vi "内置参数设置.vi"() -> ()   [LabVIEW 2016, in "斯坦道CODMn新电路板.lvlib"]
uses:
  <vilib>/Utility/miscctls.llb/LVPointTypeDef.ctl
panel:
  in  "滴定延时时间:\n(单位:毫秒)":u16
  in  "斜率阈值:":dbl
  in  "阀配置:":u8(ring) items=["三通阀", "排阀"]
  in  "AB跨度告警值:":u16
  in  "B值告警上限值:":u16
  in  "B值范围:":u16
  in  "A值告警上限值:":u16
  in  "A值范围:":u16
  in  "是否存在液位检测板:":u16(ring) items=["否", "是"]
  in  "检出限(mg/L):":dbl
  in  "测量精度(mg/L):":dbl
  in  "ILimitDown":dbl
  in  "ILimitUp:":dbl
  in  "K d:":dbl
  in  "K i:":dbl
  in  "K p:":dbl
  in  "加热超时时间:(单位:秒)":dbl
  in  "告警温度:":dbl
  in  "加热温度:  校准参数":dbl
  in  "运行速度:  (修改需要重启)":u16
  in  "偏心轮: 校准参数":dbl
  in  "注射泵加热超时时间(s):":u16
  in  "注射泵保温温度H:":u8
  in  "注射泵\n保温温度L:":u8
  in  "传感器阈值:":u16
  in  "纯水通道:":u16
  in  "滴定速度:":u16
  in  "出样速度:":u16
  in  "进样速度:":u16
  in  "阀数量:":u8(ring) items=["9通"=9, "12通"=12]
  in  "注射泵型号":u8(ring) items=["TECAN", "润泽", "旋转阀"]
  in  "阈值(高→低)(mg/L):":dbl
  in  "阈值(低→高)(mg/L):":dbl
  in  "检测下限(mg/L):":dbl
  in  "检测上限(mg/L):":dbl
  in  "关闭":bool
  in  "保存":bool
  in  "读取":bool
  # "仪器内部参数设置"
  # "~"
  # "~"
  # "~"
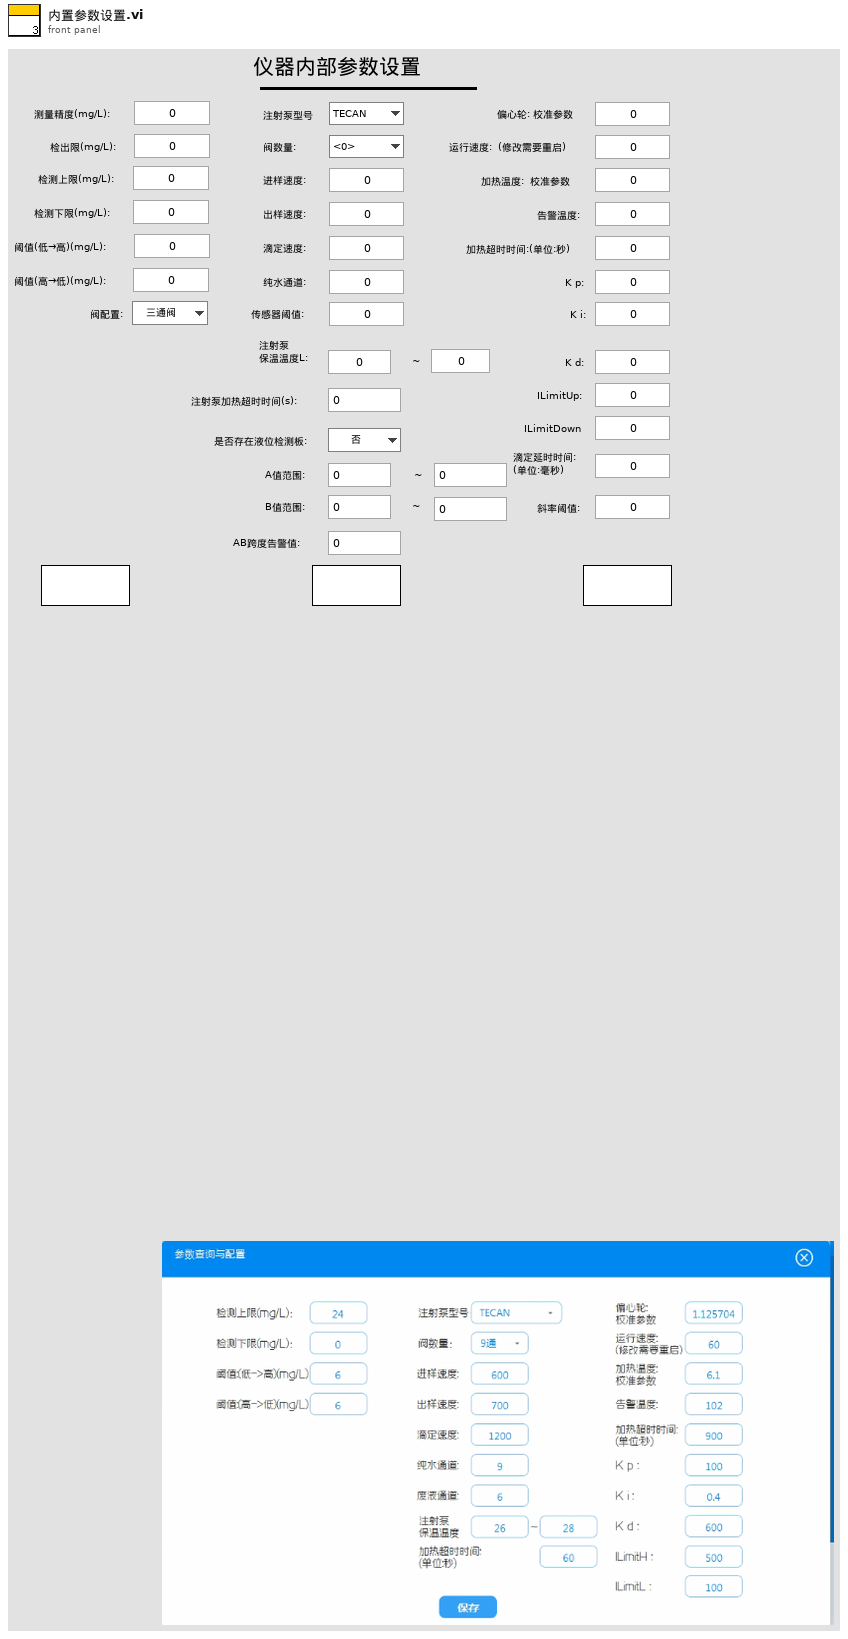
[diagram p1: front panel]
types:
  T1 = typedef "LVPointTypeDef.ctl" = cluster{"Horizontal":i16, "Vertical":i16}
  T2 = cluster{"偏心轮校准参数":dbl, "运行速度(修改需要重启)":u16, "加热温度(校准参数) ":dbl, "告警温度":dbl, "加热超时时间:(单位/秒)":dbl, "K p":dbl, "K i":dbl, "K d":dbl, "ILimitUp":dbl, "ILimitDown":dbl}
  T3 = cluster{"泵类型":u8, "阀数量":u8, "纯水通道":u16, "废液通道":u8, "进样速度":u16, "出样速度":u16, "滴定速度":u16, "注射泵保温温度L":u8, "注射泵保温温度H":u8, "注射泵加热超时时间":u16, "是否存在液位检测板":u16, "A值告警下限值":u16, "A值告警上限值":u16, "B值告警下限值":u16, "B值告警上限值":u16, "AB跨度告警值":u16, "阀配置:":u8, "滴定等待时间":u16, "滴定吸光度斜率":dbl, "传感器阈值":u16}
  T4 = cluster{"检出限":dbl, "测量精度":dbl, "上限":dbl, "下限":dbl, "阈值（低->高）":dbl, "阈值（高->低）":dbl}
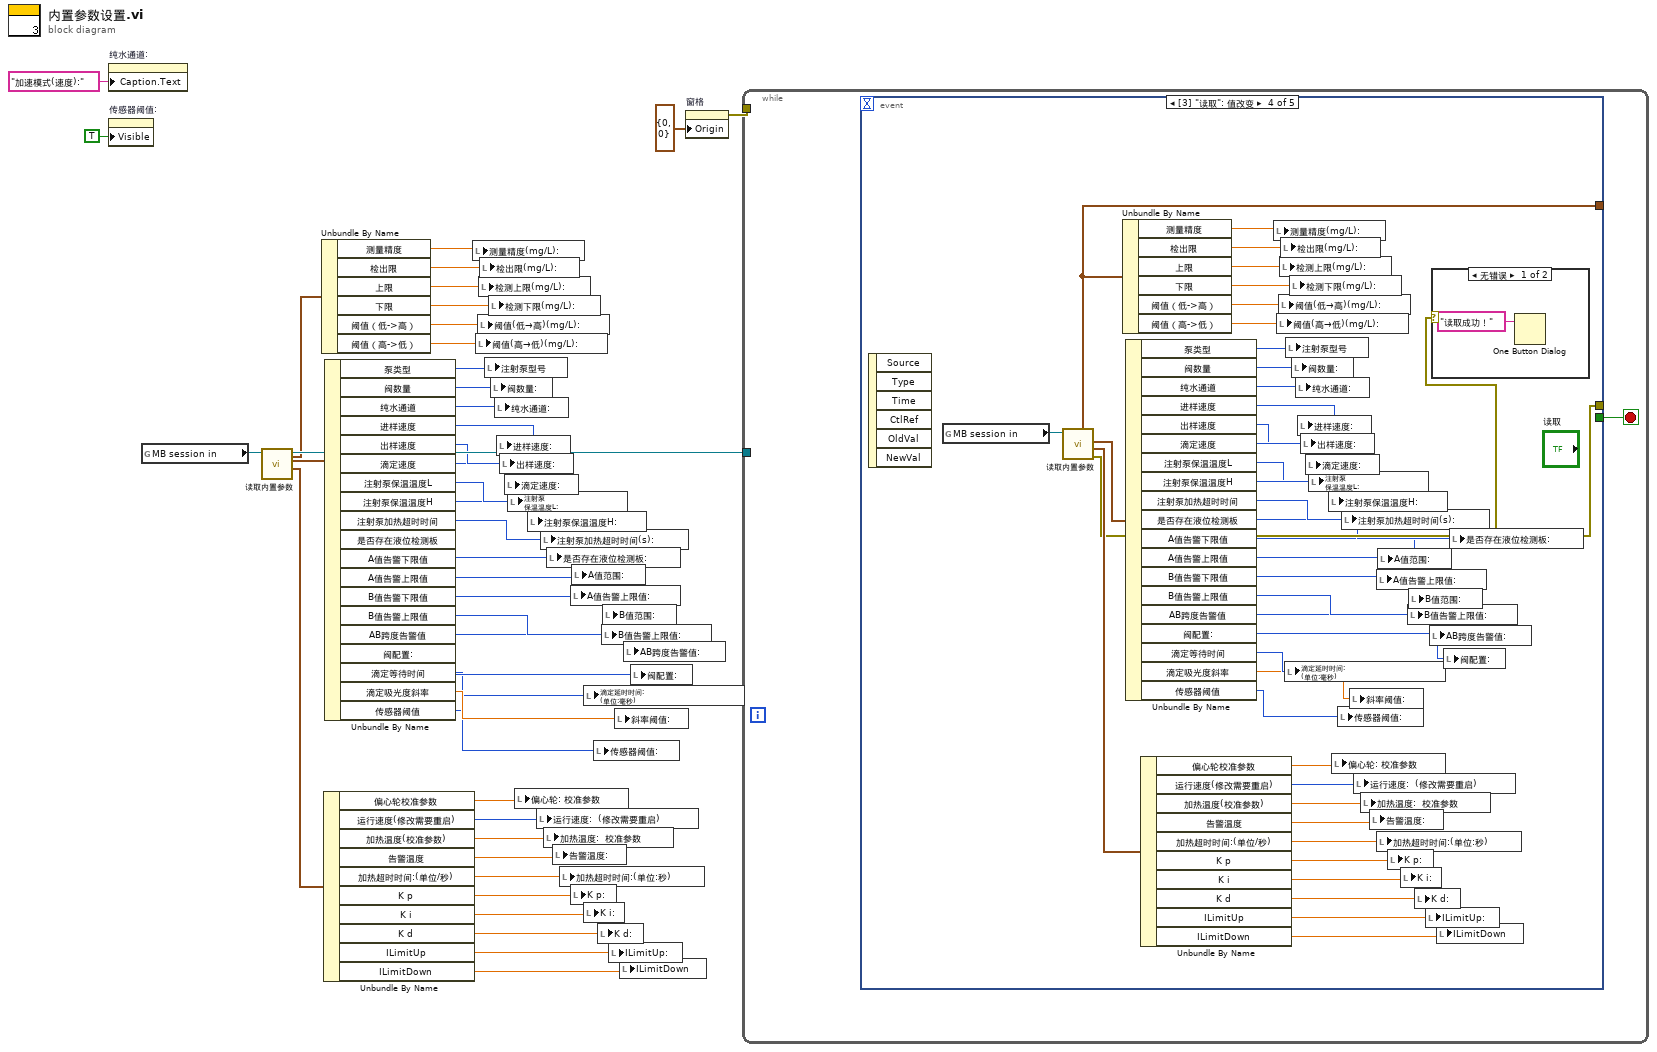
[diagram p0: block diagram]
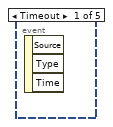
[diagram p2: hidden frame]
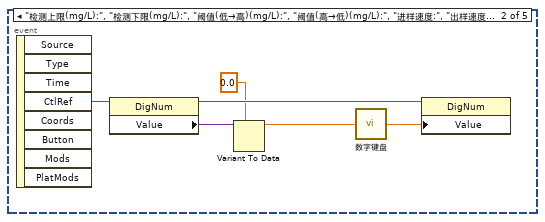
[diagram p3: hidden frame]
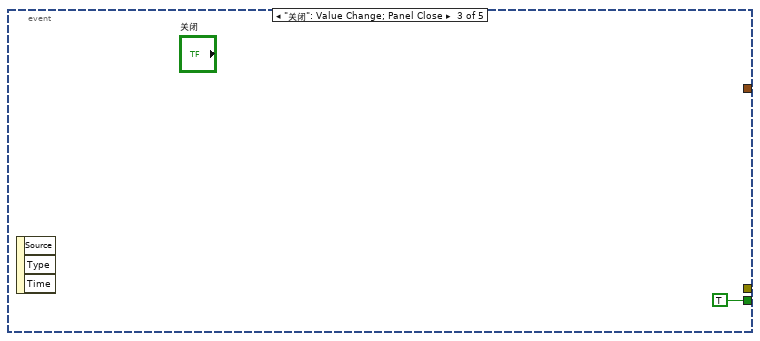
[diagram p4: hidden frame]
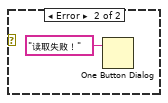
[diagram p5: hidden frame]
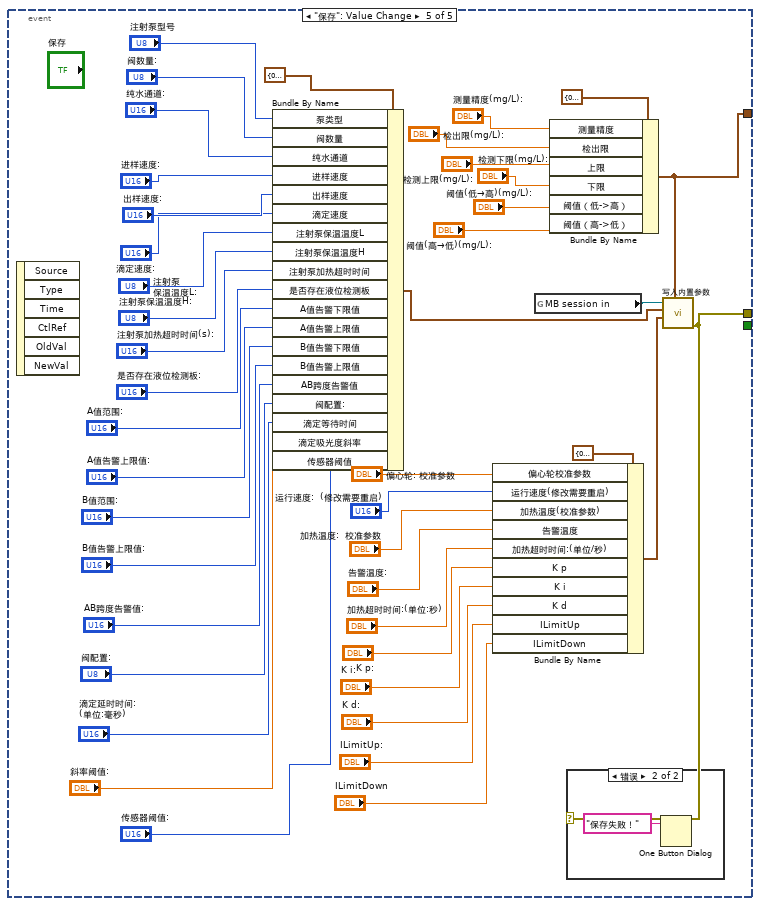
[diagram p6: hidden frame]
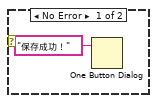
[diagram p7: hidden frame]
diagram:
  n1 = property on="纯水通道:" class="DigNum (严格)"("Caption.Text"="加速模式(速度):" ("标题.文本")) -> ()  [unwired: 2 in, 2 out]
  n2 = property on="传感器阈值:" class="DigNum (严格)"("Visible"=TRUE ("可见")) -> ()  [unwired: 2 in, 2 out]
  n3 = global read "VARCODMn全局变量.vi" "MB session in"() -> (w42:refnum<class "MB_Master.lvclass">)
  n4 = call "读取内置参数.vi"("MB session in"=w42) -> ("float"=w39:T2, "外设配置"=w40:T3, "MB session out"=w41:refnum<class "MB_Master.lvclass">, "量程参数读取"=w6:T4)  [unwired: 6 in, 1 out]
  n5 = Unbundle By Name(w6) -> ("测量精度"=w38:dbl, "检出限"=w37:dbl, "上限"=w36:dbl, "下限"=w35:dbl, "阈值（低->高）"=w34:dbl, "阈值（高->低）"=w33:dbl)
  n6 = Unbundle By Name(w39) -> ("偏心轮校准参数"=w23:dbl, "运行速度(修改需要重启)"=w22:u16, "加热温度(校准参数)"=w21:dbl, "告警温度"=w20:dbl, "加热超时时间:(单位/秒)"=w19:dbl, "K p"=w18:dbl, "K i"=w17:dbl, "K d"=w16:dbl, "ILimitUp"=w15:dbl, "ILimitDown"=w14:dbl)
  n7 = Unbundle By Name(w40) -> ("泵类型"=w32:u8, "阀数量"=w31:u8, "纯水通道"=w30:u16, "进样速度"=w29:u16, "出样速度"=w28:u16, "滴定速度"=w27:u16, "注射泵保温温度L"=w26:u8, "注射泵保温温度H"=w25:u8, "注射泵加热超时时间"=w24:u16, "是否存在液位检测板"=w13:u16, "A值告警下限值"=w12:u16, "A值告警上限值"=w11:u16, "B值告警下限值"=w10:u16, "B值告警上限值"=w9:u16, "AB跨度告警值"=w8:u16, "阀配置:"=w7:u8, "滴定等待时间"=w4:u16, "滴定吸光度斜率"=w5:dbl, "传感器阈值"=w1:u16)
  n8 = local write "测量精度(mg/L):"(w38) -> ()
  n9 = local write "阈值(高→低)(mg/L):"(w33) -> ()
  n10 = local write "阈值(低→高)(mg/L):"(w34) -> ()
  n11 = local write "检测上限(mg/L):"(w36) -> ()
  n12 = local write "检出限(mg/L):"(w37) -> ()
  n13 = local write "注射泵型号"(w32) -> ()
  n14 = local write "检测下限(mg/L):"(w35) -> ()
  n15 = local write "阀数量:"(w31) -> ()
  n16 = local write "纯水通道:"(w30) -> ()
  n17 = local write "进样速度:"(w29) -> ()
  n18 = local write "出样速度:"(w28) -> ()
  n19 = local write "滴定速度:"(w27) -> ()
  n20 = local write "注射泵\n保温温度L:"(w26) -> ()
  n21 = local write "偏心轮: 校准参数"(w23) -> ()
  n22 = local write "注射泵保温温度H:"(w25) -> ()
  n23 = local write "运行速度:  (修改需要重启)"(w22) -> ()
  n24 = local write "注射泵加热超时时间(s):"(w24) -> ()
  n25 = local write "加热温度:  校准参数"(w21) -> ()
  n26 = local write "是否存在液位检测板:"(w13) -> ()
  n27 = local write "告警温度:"(w20) -> ()
  n28 = local write "加热超时时间:(单位:秒)"(w19) -> ()
  n29 = local write "A值告警上限值:"(w11) -> ()
  n30 = local write "K p:"(w18) -> ()
  n31 = local write "A值范围:"(w12) -> ()
  n32 = local write "滴定延时时间:\n(单位:毫秒)"(w4) -> ()
  n33 = local write "K i:"(w17) -> ()
  n34 = local write "传感器阈值:"(w1) -> ()
  n35 = local write "K d:"(w16) -> ()
  n36 = local write "B值告警上限值:"(w9) -> ()
  n37 = local write "B值范围:"(w10) -> ()
  n38 = local write "ILimitUp:"(w15) -> ()
  n39 = local write "斜率阈值:"(w5) -> ()
  n40 = local write "ILimitDown"(w14) -> ()
  n41 = local write "AB跨度告警值:"(w8) -> ()
  n42 = local write "阀配置:"(w7) -> ()
  n43 = property on="窗格" class="Pane"("Origin"=T1 {"Horizontal"=0, "Vertical"=0} ("原点")) -> (error out=w43:errorcluster)  [unwired: 2 in, 1 out]
  n44 = while {
    tunnel: w43 -> [_]
    tunnel: w41 -> [_]
    stop <- w45 stop-if-true
    n45 = event shown="[3] \"读取\": 值改变" {
      selector: _ -> [_ _ _ _ _]
      dyn-events: _ -> [_ _ _ _ _]
      timeout: _ -> [_ _ _ _ _]
      tunnel: [_ _ TRUE _ _] -> w45
      tunnel: [_ _ _ w64 w109] -> _
      tunnel: [_ _ _ w56 w100] -> _
      event Timeout {
        n46 = event-data() -> ()  [unwired: 1 in, 3 out]
      }
      event "检测上限(mg/L):", "检测下限(mg/L):", "阈值(低→高)(mg/L):", "阈值(高→低)(mg/L):", "进样速度:", "出样速度:", "滴定速度:", "纯水通道:", "传感器阈值:", "注射泵\n保温温度L:", "注射泵保温温度H:", "注射泵加热超时时间(s):", "偏心轮: 校准参数", "运行速度:  (修改需要重启)", "告警温度:", "加热温度:  校准参数", "K p:", "K i:", "K d:", "ILimitUp:", "ILimitDown", "测量精度(mg/L):", "检出限(mg/L):", "A值范围:", "A值告警上限值:", "B值范围:", "B值告警上限值:", "AB跨度告警值:", "斜率阈值:", "滴定延时时间:\n(单位:毫秒)": Mouse Down {
        n47 = event-data() -> ("CtlRef"=w51:refnum<vi>)  [unwired: 1 in, 7 out]
        n48 = property class="DigNum"(reference=w51) -> (reference out=w50:refnum<vi>, "Value"=w48:variant)  [unwired: 1 in, 1 out]
        n49 = Variant To Data(type=0.0 ("OldNumber"), Variant=w48) -> (data=w46:dbl)  [unwired: 1 in, 1 out]
        n50 = call "数字键盘.vi"("OldNumber"=w46) -> ("NewNumber"=w49:dbl)
        n51 = property class="DigNum"(reference=w50, "Value"=w49) -> ()  [unwired: 1 in, 2 out]
      }
      event "关闭": Value Change; Panel Close {
        n52 = event-data() -> ()  [unwired: 1 in, 3 out]
      }
      event "读取": Value Change {
        n53 = event-data() -> ()  [unwired: 1 in, 6 out]
        n54 = global read "VARCODMn全局变量.vi" "MB session in"() -> (w65:refnum<class "MB_Master.lvclass">)
        n55 = call "读取内置参数.vi"("MB session in"=w65) -> ("error out"=w64:errorcluster, "float"=w67:T2, "外设配置"=w66:T3, "量程参数读取"=w56:T4)  [unwired: 6 in, 1 out]
        n56 = Unbundle By Name(w56) -> ("测量精度"=w68:dbl, "检出限"=w69:dbl, "上限"=w70:dbl, "下限"=w71:dbl, "阈值（低->高）"=w72:dbl, "阈值（高->低）"=w73:dbl)
        n57 = Unbundle By Name(w66) -> ("泵类型"=w74:u8, "阀数量"=w75:u8, "纯水通道"=w76:u16, "进样速度"=w77:u16, "出样速度"=w78:u16, "滴定速度"=w79:u16, "注射泵保温温度L"=w80:u8, "注射泵保温温度H"=w81:u8, "注射泵加热超时时间"=w82:u16, "是否存在液位检测板"=w63:u16, "A值告警下限值"=w62:u16, "A值告警上限值"=w61:u16, "B值告警下限值"=w60:u16, "B值告警上限值"=w59:u16, "AB跨度告警值"=w58:u16, "阀配置:"=w57:u8, "滴定等待时间"=w55:u16, "滴定吸光度斜率"=w54:dbl, "传感器阈值"=w53:u16)
        n58 = Unbundle By Name(w67) -> ("偏心轮校准参数"=w83:dbl, "运行速度(修改需要重启)"=w84:u16, "加热温度(校准参数)"=w85:dbl, "告警温度"=w86:dbl, "加热超时时间:(单位/秒)"=w87:dbl, "K p"=w88:dbl, "K i"=w89:dbl, "K d"=w90:dbl, "ILimitUp"=w91:dbl, "ILimitDown"=w92:dbl)
        n59 = local write "测量精度(mg/L):"(w68) -> ()
        n60 = local write "阈值(高→低)(mg/L):"(w73) -> ()
        n61 = local write "阈值(低→高)(mg/L):"(w72) -> ()
        n62 = local write "检测上限(mg/L):"(w70) -> ()
        n63 = local write "检出限(mg/L):"(w69) -> ()
        n64 = local write "滴定延时时间:\n(单位:毫秒)"(w55) -> ()
        n65 = local write "注射泵型号"(w74) -> ()
        n66 = local write "检测下限(mg/L):"(w71) -> ()
        n67 = local write "阀数量:"(w75) -> ()
        n68 = local write "纯水通道:"(w76) -> ()
        n69 = local write "进样速度:"(w77) -> ()
        n70 = local write "出样速度:"(w78) -> ()
        n71 = local write "滴定速度:"(w79) -> ()
        n72 = local write "注射泵\n保温温度L:"(w80) -> ()
        n73 = local write "注射泵保温温度H:"(w81) -> ()
        n74 = local write "偏心轮: 校准参数"(w83) -> ()
        n75 = local write "传感器阈值:"(w53) -> ()
        n76 = local write "注射泵加热超时时间(s):"(w82) -> ()
        n77 = local write "斜率阈值:"(w54) -> ()
        n78 = local write "运行速度:  (修改需要重启)"(w84) -> ()
        n79 = local write "加热温度:  校准参数"(w85) -> ()
        n80 = local write "告警温度:"(w86) -> ()
        n81 = local write "A值告警上限值:"(w61) -> ()
        n82 = local write "加热超时时间:(单位:秒)"(w87) -> ()
        n83 = local write "A值范围:"(w62) -> ()
        n84 = local write "K p:"(w88) -> ()
        n85 = local write "K i:"(w89) -> ()
        n86 = local write "B值告警上限值:"(w59) -> ()
        n87 = local write "B值范围:"(w60) -> ()
        n88 = local write "K d:"(w90) -> ()
        n89 = local write "ILimitUp:"(w91) -> ()
        n90 = local write "AB跨度告警值:"(w58) -> ()
        n91 = case shown="无错误" w64 {
          frame No Error {
            n92 = One Button Dialog(message="读取成功！" ("消息")) -> ()  [unwired: 1 in, 1 out]
          }
          frame Error {
            n93 = One Button Dialog(message="读取失败！" ("消息")) -> ()  [unwired: 1 in, 1 out]
          }
        }
        n94 = local write "ILimitDown"(w92) -> ()
        n95 = local write "阀配置:"(w57) -> ()
        n96 = local write "是否存在液位检测板:"(w63) -> ()
      }
      event "保存": Value Change {
        n97 = event-data() -> ()  [unwired: 1 in, 6 out]
        n98 = Bundle By Name(cluster=T3 {"泵类型"=0, "阀数量"=0, "纯水通道"=0, "废液通道"=0, "进样速度"=0, "出样速度"=0, "滴定速度"=0, "注射泵保温温度L"=0, "注射泵保温温度H"=0, "注射泵加热超时时间"=0, "是否存在液位检测板"=0, "A值告警下限值"=0, "A值告警上限值"=0, "B值告警下限值"=0, "B值告警上限值"=0, "AB跨度告警值"=0, "阀配置:"=0, "滴定等待时间"=0, "滴定吸光度斜率"=0.0, "传感器阈值"=0} ("外设配置"), "泵类型"="注射泵型号", "阀数量"="阀数量:", "纯水通道"="纯水通道:", "进样速度"="进样速度:", "出样速度"="出样速度:", "滴定速度"="滴定速度:", "注射泵保温温度L"="注射泵\n保温温度L:", "注射泵保温温度H"="注射泵保温温度H:", "注射泵加热超时时间"="注射泵加热超时时间(s):", "是否存在液位检测板"="是否存在液位检测板:", "A值告警下限值"="A值范围:", "A值告警上限值"="A值告警上限值:", "B值告警下限值"="B值范围:", "B值告警上限值"="B值告警上限值:", "AB跨度告警值"="AB跨度告警值:", "阀配置:"="阀配置:", "滴定等待时间"="滴定延时时间:\n(单位:毫秒)", "滴定吸光度斜率"="斜率阈值:", "传感器阈值"="传感器阈值:") -> (w97:T3)
        n99 = Bundle By Name(cluster=T2 {"偏心轮校准参数"=0.0, "运行速度(修改需要重启)"=0, "加热温度(校准参数) "=0.0, "告警温度"=0.0, "加热超时时间:(单位/秒)"=0.0, "K p"=0.0, "K i"=0.0, "K d"=0.0, "ILimitUp"=0.0, "ILimitDown"=0.0} ("float"), "偏心轮校准参数"="偏心轮: 校准参数", "运行速度(修改需要重启)"="运行速度:  (修改需要重启)", "加热温度(校准参数)"="加热温度:  校准参数", "告警温度"="告警温度:", "加热超时时间:(单位/秒)"="加热超时时间:(单位:秒)", "K p"="K p:", "K i"="K i:", "K d"="K d:", "ILimitUp"="ILimitUp:", "ILimitDown"="ILimitDown") -> (w110:T2)
        n100 = global read "VARCODMn全局变量.vi" "MB session in"() -> (w137:refnum<class "MB_Master.lvclass">)
        n101 = Bundle By Name(cluster=T4 {"检出限"=0.0, "测量精度"=0.0, "上限"=0.0, "下限"=0.0, "阈值（低->高）"=0.0, "阈值（高->低）"=0.0} ("量程参数读取"), "测量精度"="测量精度(mg/L):", "检出限"="检出限(mg/L):", "上限"="检测上限(mg/L):", "下限"="检测下限(mg/L):", "阈值（低->高）"="阈值(低→高)(mg/L):", "阈值（高->低）"="阈值(高→低)(mg/L):") -> (w100:T4)
        n102 = call "写入内置参数.vi"("量程参数读取"=w100, "float"=w110, "外设配置"=w97, "MB session in"=w137) -> ("error out"=w109:errorcluster)  [unwired: 6 in, 1 out]
        n103 = case shown="错误" w109 {
          frame No Error {
            n104 = One Button Dialog(message="保存成功！" ("消息")) -> ()  [unwired: 1 in, 1 out]
          }
          frame Error {
            n105 = One Button Dialog(message="保存失败！" ("消息")) -> ()  [unwired: 1 in, 1 out]
          }
        }
      }
    }
  }
